vi "acknowledgeIRQ.vi"(8 "error in (no error)":errorcluster, 10 "IRQs":i32[](array[numeric]), 11 "FPGA in":refnum<class "FPGA.lvclass">) -> (0 "error out":errorcluster, 3 "FPGA out":refnum<class "FPGA.lvclass">)   [LabVIEW 2016, in "FPGA.lvclass"]
uses:
  FPGA.lvclass
  FPGA.lvclass/FPGA.ctl
  <vilib>/Utility/error.llb/Error Cluster From Error Code.vi
  <vilib>/rvi/interface/nirviMethod/nirviMethod.xnode
  <vilib>/FPGAPlugInAG/Dynamic/niLvFpga_AcknowledgeIrq_Dynamic.vi
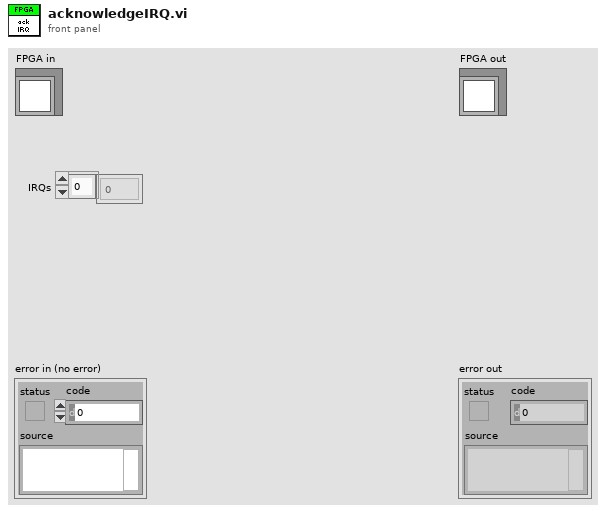
[diagram p1: front panel]
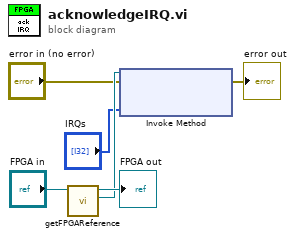
[diagram p0: block diagram]
diagram:
  n1 = call "getFPGAReference.vi"("FPGA in"="FPGA in") -> ("FPGAReference"=w4:refnum<k20>, "FPGA out"=→"FPGA out":refnum<class "FPGA.lvclass">)  [unwired: 9 in]
  n2 = xnode "Invoke Method"("FPGA VI Reference In"=w4, "error in"="error in (no error)", "IRQ Number(s)"="IRQs") -> ("error out"=→"error out":errorcluster)  [unwired: 1 out]
